vi "G#SubTemplateG3_SetModifiedClassAttributes.vi"(0 "reference in":refnum<class "G#SubTemplateG3.lvclass">, 2 "attributes":T1, 3 "Only unlock data? (F)":bool, 4 "Unlock data if error? (T)":bool=TRUE, 5 "error in (no error)":errorcluster, 7 "Update data even if error? (F)":bool) -> (14 "reference out":refnum<class "G#SubTemplateG3.lvclass">, 19 "error out":errorcluster)   [LabVIEW 2020, in "G#SubTemplateG3.lvclass"]
doc: "This VI overwrites the attributes associated with the object reference and unlocks it for write access. If error in is set, the object is unlocked but its data will not be modified.\n\nIn order to use this VI, you must first successfully lock the object's data using this class GetAttributesToModify VI."
uses:
  <vilib>/addons/_AddQ/G#Templates/G#SubTemplateG3/G#SubTemplateG3.lvclass
  <vilib>/addons/_AddQ/G#Templates/G#SubTemplateG3/protected/ClassAttributes.ctl
  <vilib>/addons/_AddQ/G#Templates/G#BaseTemplateG3/protected/ClassAttributes.ctl
  <vilib>/addons/_AddQ/G#Templates/G#SubTemplateG3/G#SubTemplateG3.lvclass/G#SubTemplateG3.ctl
  <vilib>/addons/_AddQ/G#Templates/G#BaseTemplateG3/G#BaseTemplateG3.lvclass
  C:/Program Files (x86)/National Instruments/LabVIEW 2020/vi.lib/addons/_AddQ/G#Templates/G#BaseTemplateG3/G#BaseTemplateG3.lvclass
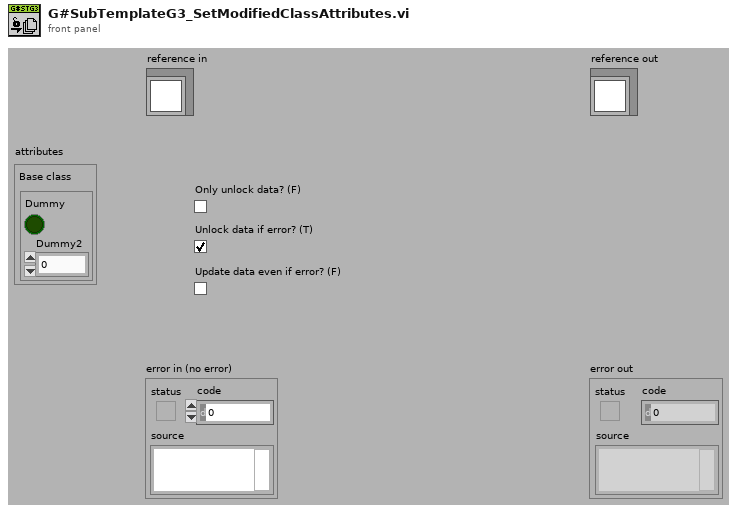
[diagram p1: front panel]
types:
  T1 = typedef "G#SubTemplateG3.lvclass/ClassAttributes.ctl" = cluster{"Base class":T2}
  T2 = typedef "G#BaseTemplateG3.lvclass/ClassAttributes.ctl" = cluster{"Dummy":bool, "Dummy2":dbl}
  T3 = typedef "G#SubTemplateG3.lvclass/ClassAttributesRef.ctl" = refnum<data-value>
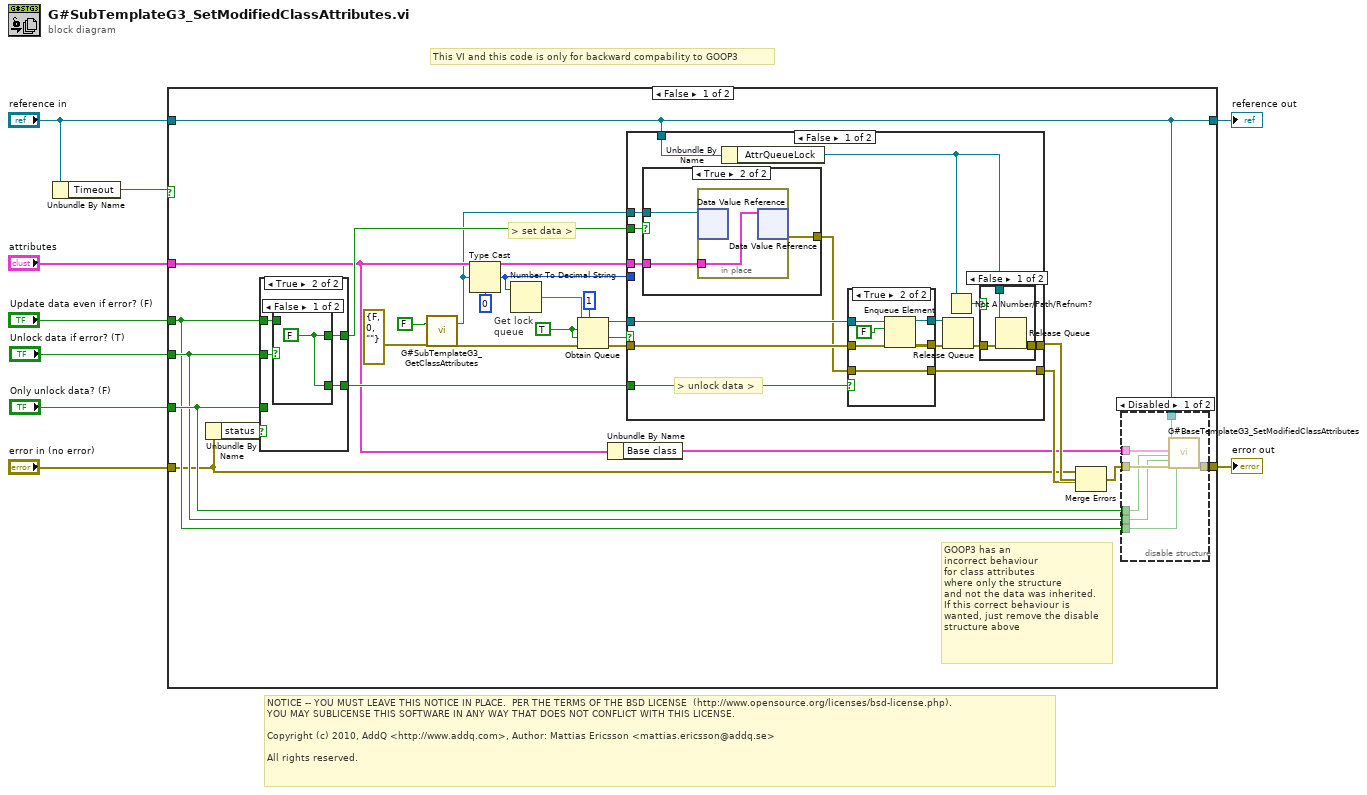
[diagram p0: block diagram]
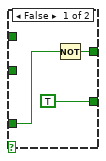
[diagram p3: hidden frame]
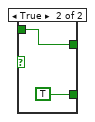
[diagram p4: hidden frame]
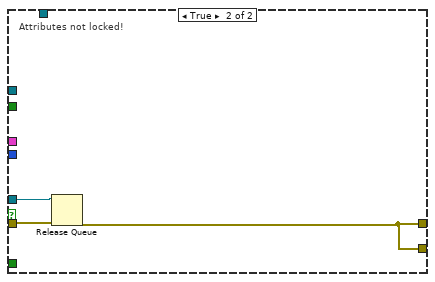
[diagram p8: hidden frame]
diagram:
  # "NOTICE -- YOU MUST LEAVE THIS NOTICE IN PLACE.  PER THE TERMS OF THE BSD LICENSE  (http://www.opensource.org/licenses/bsd-license.php).\nYOU MAY SUBLICENSE THIS SOFTWARE IN ANY WAY THAT DOES NOT CONFLICT WITH THIS LICENSE.\n\nCopyright (c) 2010, AddQ <http://www.addq.com>, Author: Mattias Ericsson <mattias.ericsson@addq.se>\n\nAll rights reserved."
  # "This VI and this code is only for backward compability to GOOP3"
  n1 = Unbundle By Name("reference in") -> ("Timeout"=w1:bool)
  n2 = case shown="False" w1 {
    tunnel: [w21 w89] -> w9
    tunnel: "reference in" -> [w20 w90]
    tunnel: "error in (no error)" -> [w12 w89]
    tunnel: "attributes" -> [w19 _]
    tunnel: "Only unlock data? (F)" -> [w17 _]
    tunnel: "Unlock data if error? (T)" -> [w16 _]
    tunnel: "Update data even if error? (F)" -> [w15 _]
    tunnel: [w20 w90] -> w2
    frame False {
      w34 = TRUE ("create if not found? (T)")
      # "GOOP3 has an\nincorrect behaviour\nfor class attributes\nwhere only the structure\nand not the data was inherited.\nIf this correct behaviour is\nwanted, just remove the disable\nstructure above"
      # "Get lock\nqueue"
      # "> set data >"
      n3 = Unbundle By Name(w12) -> ("status"=w28:bool)
      n4 = case shown="True" w28 {
        tunnel: [w44 w49] -> w27
        tunnel: w17 -> [w46 _]
        tunnel: [TRUE w48] -> w26
        tunnel: w16 -> [_ w50]
        tunnel: w15 -> [_ w47]
        frame False {
          n5 = Not(x=w46) -> (.not. x?=w44:bool)
        }
        frame True {
          n6 = case shown="False" w50 {
            tunnel: [w51 w52] -> w49
            tunnel: [w51 TRUE] -> w48
            tunnel: w47 -> [_ w52]
            frame False {
              w51 = FALSE
            }
            frame True {
            }
          }
        }
      }
      n7 = call <vilib>:"G#SubTemplateG3_GetClassAttributes.vi"("return data? (T)"=FALSE ("return data"), "error in (no error)"=errorcluster {"status"=FALSE, "code"=0, "source"=""}) -> ("class attributes ref"=w13:T3, "error out"=w11:errorcluster)  [unwired: 13 in, 3 out]
      n8 = Type Cast(type=u32 0, x=w13) -> (*(type *) &x=w24:u32)
      n9 = Number To Decimal String(number=w24) -> (decimal integer string=w35:string)  [unwired: 1 in]
      n10 = Obtain Queue(max queue size (-1, unlimited)=1, name (unnamed)=w35, element data type=w34, create if not found? (T)=w34, error in (no error)=w11) -> (queue out=w30:refnum<queue>, created new?=w31:bool, error out=w32:errorcluster)
      n11 = Unbundle By Name(w19) -> ("Base class"=w18:T2)
      n12 = case shown="False" w31 {
        tunnel: w32 -> [w68 w87]
        tunnel: w30 -> [w67 w86]
        tunnel: [w61 w88] -> w29
        tunnel: w24 -> [_ _]
        tunnel: w27 -> [w64 _]
        tunnel: w19 -> [w63 _]
        tunnel: w26 -> [w62 _]
        tunnel: w20 -> [w59 _]
        tunnel: [w57 w88] -> w23
        tunnel: w13 -> [w56 _]
        frame False {
          # "> unlock data >"
          n13 = case shown="True" w64 {
            tunnel: w63 -> [_ w84]
            tunnel: [_ w83] -> w58
            tunnel: w56 -> [_ w82]
            frame False {
            }
            frame True {
              n14 = in-place {
                in-place-border: w84 -> [w85]
                n15 = in-place-dvr #1(w82) -> ()  [unwired: 2 out]
                n16 = in-place-dvr #1(w85) -> (w83:errorcluster)  [unwired: 1 out]
              }
            }
          }
          n17 = Unbundle By Name(w59) -> ("AttrQueueLock"=w55:refnum<queue>)
          n18 = case shown="True" w62 {
            tunnel: w68 -> [w74 w81]
            tunnel: w67 -> [w75 w80]
            tunnel: [w74 w79] -> w66
            tunnel: [w75 w78] -> w65
            tunnel: w58 -> [w73 w76]
            tunnel: [w73 w76] -> w57
            frame False {
            }
            frame True {
              n19 = Enqueue Element(queue=w80, element=FALSE, error in (no error)=w81) -> (queue out=w78:refnum<queue>, error out=w79:errorcluster)  [unwired: 1 in, 1 out]
            }
          }
          n20 = Release Queue(queue=w65, error in (no error)=w66) -> (error out=w60:errorcluster)  [unwired: 1 in, 2 out]
          n21 = Not A Number/Path/Refnum?(number/path/refnum=w55) -> (NaN/Path/Refnum?=w54:bool)
          n22 = case shown="False" w54 {
            tunnel: [w71 w72] -> w61
            tunnel: w60 -> [w70 w72]
            tunnel: w55 -> [w69 _]
            frame False {
              n23 = Release Queue(queue=w69, error in (no error)=w70) -> (error out=w71:errorcluster)  [unwired: 1 in, 2 out]
            }
            frame True {
            }
          }
        }
        frame True {
          # "Attributes not locked!"
          n24 = Release Queue(queue=w86, error in (no error)=w87) -> (error out=w88:errorcluster)  [unwired: 1 in, 2 out]
        }
      }
      n25 = Merge Errors(w12, w29, w23) -> (w22:errorcluster)
      n26 = disable-structure shown="Disabled" {
        disable-tunnel: w22 -> [w42 w43]
        disable-tunnel: [w41 w43] -> w21
        disable-tunnel: w20 -> [w40 _]
        disable-tunnel: w18 -> [w39 _]
        disable-tunnel: w17 -> [w38 _]
        disable-tunnel: w16 -> [w37 _]
        disable-tunnel: w15 -> [w36 _]
        frame Disabled {
          n27 = call <vilib>:"G#BaseTemplateG3_SetModifiedClassAttributes.vi"("reference in"=w40, "attributes"=w39, "Only unlock data? (F)"=w38, "Unlock data if error? (T)"=w37, "error in (no error)"=w42, "Update data even if error? (F)"=w36) -> ("error out"=w41:errorcluster)  [unwired: 12 in, 1 out]
        }
        frame Enabled {
        }
      }
    }
    frame True {
      # "Timeout or not locked!"
    }
  }
  "error out" <- w9
  "reference out" <- w2
